vi "OE2012&OE2022_Configure Auxout.vi"(7 "OE2012&OE2022_\nConfigure Auxout":T1={"Offset(%)"=0.0, "Expand"=1, "Source"=3, "Aux Output"=1, "Sensitivity "=24, "DC Voltage"=0.0} {"DC Voltage" min=-100.0 max=100.0 format="%#.2g"; "Sensitivity" items=["1 nV/fA", "2 nV/fA", "5 nV/fA", "10 nV/fA", "20 nV/fA", "50 nV/fA", "100 nV/fA", "200 nV/fA", "500 nV/fA", "1 uV/pA", "2 uV/pA", "5 uV/pA", "10 uV/pA", "20 uV/pA", "50 uV/pA", "100 uV/pA", "200 uV/pA", "500 uV/pA", "1 mV/nA", "2 mV/nA", "5 mV/nA", "10 mV/nA", "20 mV/nA", "50 mV/nA", "100 mV/nA", "200 mV/nA", "500 mV/nA", "1 V/uA", "2 V/uA", "5 V/uA"]; "Aux Output" items=["AUX1"=1, "AUX2"=2, "AUX3"=3, "AUX4"=4]; "Source" items=["DC OUT", "X-Demod1", "Y-Demod1", "R-Demod1", "Theta-Demod1", "X-Demod2", "Y-Demod2", "R-Demod2", "Theta-Demod2", "X-Demod3", "Y-Demod3", "R-Demod3", "Theta-Demod3", "X-Demod4", "Y-Demod4", "R-Demod4", "Theta-Demod4", "X-Demod5", "Y-Demod5", "R-Demod5", "Theta-Demod5", "X-Demod6", "Y-Demod6", "R-Demod6", "Theta-Demod6", "X-Demod7", "Y-Demod7", "R-Demod7", "Theta-Demod7", "X-Demod8", "Y-Demod8", "R-Demod8", "Theta-Demod8", "AUXIN1", "AUXIN2", "AUXIN3", "AUXIN4"]; "Expand" min=1 max=256; "Offset(%)" min=-100.0 max=100.0 format="%#.2g"}, 8 "Error in (no error)":errorcluster caption="error out（no error）", 9 "Remote Mode":u16(ring) items=["USB", "RS232", "GPIB", "Ethernet"], 11 "VISA resource name":refnum<visa-resource-name>) -> (0 "Error out":errorcluster caption="error out", 1 "Output String":string, 3 "VISA resource  out":refnum<visa-resource-name>)   [LabVIEW 2011]
panel:
  out "Connection ID out":refnum<k5>
  in  "Connection ID in":refnum<k5>
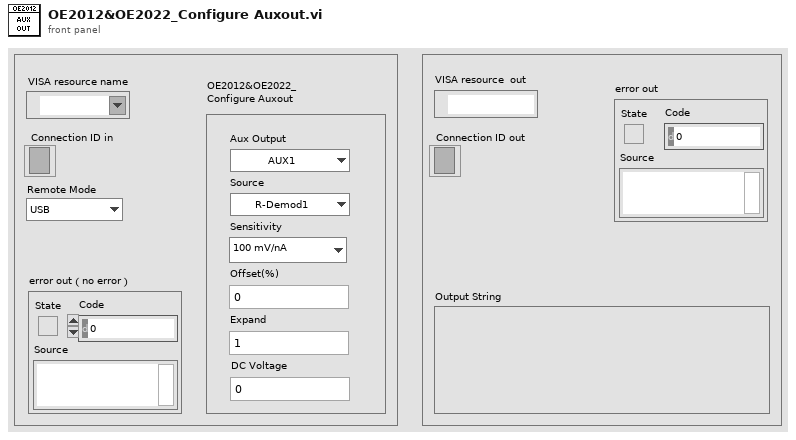
[diagram p1: front panel]
types:
  T1 = cluster{"Offset(%)":dbl, "Expand":i16, "Source":u16, "Aux Output":u16, "Sensitivity ":u16, "DC Voltage":dbl}
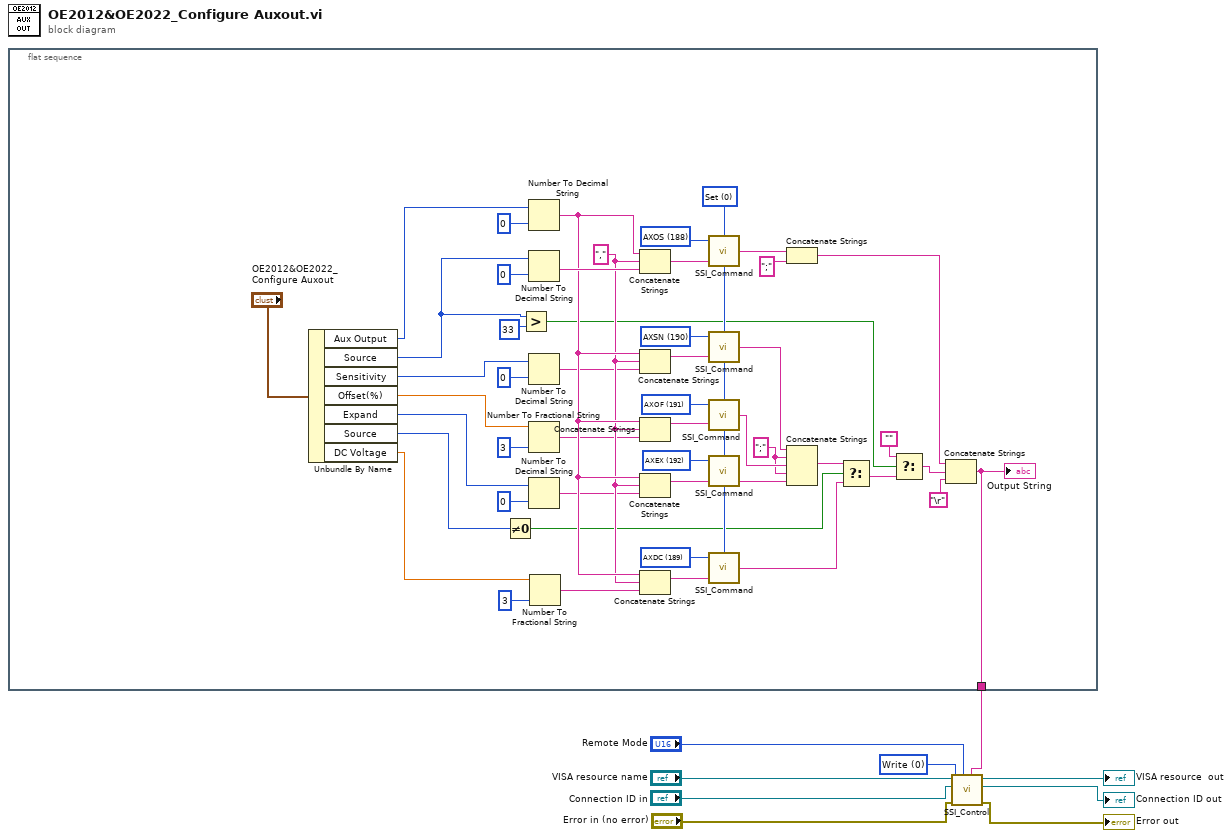
[diagram p0: block diagram]
diagram:
  w8 = u16 0 items=["Write", "Read"] ("Control")
  n1 = flat-sequence {
    tunnel: [w22] -> w1
    frame #0 {
      w10 = u16 189 items=["ISRC", "IGND", "ICPL", "ILIN", "PHAS", "FMOD", "RSLP", "FREQ", "SWPT", "SLLM", "SULM", "SSLL", "SSLG", "STLM", "SWRM", "IRNG", "SENS", "RMOD", "OFLT", "OFSL", "SYNC", "DMOD", "HARM", "DARB", "SWVT", "SLVL", "SVLL", "SVUL", "SVSL", "SVSG", "SVTM", "SVRM", "RALL", "SNAP", "OUTP", "OAUX", "COUT", "CAUX", "COFP", "CEXP", "FPOP", "OEXP", "*IDN", "*RST", "OVLD", "INOV", "GNOV", "*PLL", "SSET", "RSET", "AGAN", "APHS", "ARSV", "ASCL", "EQCD", "EQCS", "SPED", "SRAT", "SLEN", "SSLE", "STRG", "SPRM", "STRD", "PAUS", "REST", "SPTS", "TRCA", "TEMP", "RSTU", "INHZ", "DEQU", "SADD", "ARNG", "CSPE", "ISRCD", "IGNDD", "ICPLD", "ILIND", "PHASD", "FMODD", "RSLPD", "FREQD", "SWPTD", "SLLMD", "SULMD", "SSLLD", "SSLGD", "STLMD", "SWRMD", "SENSD", "RMODD", "OFLTD", "OFSLD", "SYNCD", "HARMD", "EQCDD", "EQCSD", "SNAPD", "OUTPD", "SWVTD", "SLVLD", "SVLLD", "SVULD", "SVSLD", "SVSGD", "SVTMD", "SVRMD", "SVDCD", "ARSVD", "AGAND", "APHSD", "ASCLD", "FPOPD", "CAUXD", "OEXPD", "SPEDD", "SRATD", "SLEND", "SSLED", "STRGD", "SPRMD", "STRDD", "PAUSD", "RESTD", "SPTSD", "TRCAD", "*IDND", "*RSTD", "INOVD", "GNOVD", "*PLLD", "SSETD", "RSETD", "RALLD", "NIPA", "NSMA", "NGWA", "NMAC", "NMOD", "TRIG", "TRCB", "INHZD", "ISAMD", "IRAGD", "RRAGD", "SOFFD", "DMODD", "COUTD", "COFPD", "CEXPD", "ARNGD", "OAUXD", "TRIM", "SUITD", "SNHZD", "AOFSD", "RSRC", "FEXT", "FINT", "DSRC", "DARF", "DEAF", "DREF", "SSRC", "STTL", "SIGO", "SLVL", "SOFF", "SPHS", "TPHS", "SMOD", "MARF", "AMSR", "AMDP", "FMSR", "FMDV", "PMSR", "PMDV", "CHDC", "AUXV", "AFLT", "AOFP", "DSELD", "FEMSD", "SLVTD", "SLVBD", "DMFR", "FCMB", "AXOS", "AXDC", "AXSN", "AXOF", "AXEX"] ("Command Type")
      w11 = u16 192 items=["ISRC", "IGND", "ICPL", "ILIN", "PHAS", "FMOD", "RSLP", "FREQ", "SWPT", "SLLM", "SULM", "SSLL", "SSLG", "STLM", "SWRM", "IRNG", "SENS", "RMOD", "OFLT", "OFSL", "SYNC", "DMOD", "HARM", "DARB", "SWVT", "SLVL", "SVLL", "SVUL", "SVSL", "SVSG", "SVTM", "SVRM", "RALL", "SNAP", "OUTP", "OAUX", "COUT", "CAUX", "COFP", "CEXP", "FPOP", "OEXP", "*IDN", "*RST", "OVLD", "INOV", "GNOV", "*PLL", "SSET", "RSET", "AGAN", "APHS", "ARSV", "ASCL", "EQCD", "EQCS", "SPED", "SRAT", "SLEN", "SSLE", "STRG", "SPRM", "STRD", "PAUS", "REST", "SPTS", "TRCA", "TEMP", "RSTU", "INHZ", "DEQU", "SADD", "ARNG", "CSPE", "ISRCD", "IGNDD", "ICPLD", "ILIND", "PHASD", "FMODD", "RSLPD", "FREQD", "SWPTD", "SLLMD", "SULMD", "SSLLD", "SSLGD", "STLMD", "SWRMD", "SENSD", "RMODD", "OFLTD", "OFSLD", "SYNCD", "HARMD", "EQCDD", "EQCSD", "SNAPD", "OUTPD", "SWVTD", "SLVLD", "SVLLD", "SVULD", "SVSLD", "SVSGD", "SVTMD", "SVRMD", "SVDCD", "ARSVD", "AGAND", "APHSD", "ASCLD", "FPOPD", "CAUXD", "OEXPD", "SPEDD", "SRATD", "SLEND", "SSLED", "STRGD", "SPRMD", "STRDD", "PAUSD", "RESTD", "SPTSD", "TRCAD", "*IDND", "*RSTD", "INOVD", "GNOVD", "*PLLD", "SSETD", "RSETD", "RALLD", "NIPA", "NSMA", "NGWA", "NMAC", "NMOD", "TRIG", "TRCB", "INHZD", "ISAMD", "IRAGD", "RRAGD", "SOFFD", "DMODD", "COUTD", "COFPD", "CEXPD", "ARNGD", "OAUXD", "TRIM", "SUITD", "SNHZD", "AOFSD", "RSRC", "FEXT", "FINT", "DSRC", "DARF", "DEAF", "DREF", "SSRC", "STTL", "SIGO", "SLVL", "SOFF", "SPHS", "TPHS", "SMOD", "MARF", "AMSR", "AMDP", "FMSR", "FMDV", "PMSR", "PMDV", "CHDC", "AUXV", "AFLT", "AOFP", "DSELD", "FEMSD", "SLVTD", "SLVBD", "DMFR", "FCMB", "AXOS", "AXDC", "AXSN", "AXOF", "AXEX"] ("Command Type")
      w12 = u16 191 items=["ISRC", "IGND", "ICPL", "ILIN", "PHAS", "FMOD", "RSLP", "FREQ", "SWPT", "SLLM", "SULM", "SSLL", "SSLG", "STLM", "SWRM", "IRNG", "SENS", "RMOD", "OFLT", "OFSL", "SYNC", "DMOD", "HARM", "DARB", "SWVT", "SLVL", "SVLL", "SVUL", "SVSL", "SVSG", "SVTM", "SVRM", "RALL", "SNAP", "OUTP", "OAUX", "COUT", "CAUX", "COFP", "CEXP", "FPOP", "OEXP", "*IDN", "*RST", "OVLD", "INOV", "GNOV", "*PLL", "SSET", "RSET", "AGAN", "APHS", "ARSV", "ASCL", "EQCD", "EQCS", "SPED", "SRAT", "SLEN", "SSLE", "STRG", "SPRM", "STRD", "PAUS", "REST", "SPTS", "TRCA", "TEMP", "RSTU", "INHZ", "DEQU", "SADD", "ARNG", "CSPE", "ISRCD", "IGNDD", "ICPLD", "ILIND", "PHASD", "FMODD", "RSLPD", "FREQD", "SWPTD", "SLLMD", "SULMD", "SSLLD", "SSLGD", "STLMD", "SWRMD", "SENSD", "RMODD", "OFLTD", "OFSLD", "SYNCD", "HARMD", "EQCDD", "EQCSD", "SNAPD", "OUTPD", "SWVTD", "SLVLD", "SVLLD", "SVULD", "SVSLD", "SVSGD", "SVTMD", "SVRMD", "SVDCD", "ARSVD", "AGAND", "APHSD", "ASCLD", "FPOPD", "CAUXD", "OEXPD", "SPEDD", "SRATD", "SLEND", "SSLED", "STRGD", "SPRMD", "STRDD", "PAUSD", "RESTD", "SPTSD", "TRCAD", "*IDND", "*RSTD", "INOVD", "GNOVD", "*PLLD", "SSETD", "RSETD", "RALLD", "NIPA", "NSMA", "NGWA", "NMAC", "NMOD", "TRIG", "TRCB", "INHZD", "ISAMD", "IRAGD", "RRAGD", "SOFFD", "DMODD", "COUTD", "COFPD", "CEXPD", "ARNGD", "OAUXD", "TRIM", "SUITD", "SNHZD", "AOFSD", "RSRC", "FEXT", "FINT", "DSRC", "DARF", "DEAF", "DREF", "SSRC", "STTL", "SIGO", "SLVL", "SOFF", "SPHS", "TPHS", "SMOD", "MARF", "AMSR", "AMDP", "FMSR", "FMDV", "PMSR", "PMDV", "CHDC", "AUXV", "AFLT", "AOFP", "DSELD", "FEMSD", "SLVTD", "SLVBD", "DMFR", "FCMB", "AXOS", "AXDC", "AXSN", "AXOF", "AXEX"] ("Command Type")
      w13 = u16 190 items=["ISRC", "IGND", "ICPL", "ILIN", "PHAS", "FMOD", "RSLP", "FREQ", "SWPT", "SLLM", "SULM", "SSLL", "SSLG", "STLM", "SWRM", "IRNG", "SENS", "RMOD", "OFLT", "OFSL", "SYNC", "DMOD", "HARM", "DARB", "SWVT", "SLVL", "SVLL", "SVUL", "SVSL", "SVSG", "SVTM", "SVRM", "RALL", "SNAP", "OUTP", "OAUX", "COUT", "CAUX", "COFP", "CEXP", "FPOP", "OEXP", "*IDN", "*RST", "OVLD", "INOV", "GNOV", "*PLL", "SSET", "RSET", "AGAN", "APHS", "ARSV", "ASCL", "EQCD", "EQCS", "SPED", "SRAT", "SLEN", "SSLE", "STRG", "SPRM", "STRD", "PAUS", "REST", "SPTS", "TRCA", "TEMP", "RSTU", "INHZ", "DEQU", "SADD", "ARNG", "CSPE", "ISRCD", "IGNDD", "ICPLD", "ILIND", "PHASD", "FMODD", "RSLPD", "FREQD", "SWPTD", "SLLMD", "SULMD", "SSLLD", "SSLGD", "STLMD", "SWRMD", "SENSD", "RMODD", "OFLTD", "OFSLD", "SYNCD", "HARMD", "EQCDD", "EQCSD", "SNAPD", "OUTPD", "SWVTD", "SLVLD", "SVLLD", "SVULD", "SVSLD", "SVSGD", "SVTMD", "SVRMD", "SVDCD", "ARSVD", "AGAND", "APHSD", "ASCLD", "FPOPD", "CAUXD", "OEXPD", "SPEDD", "SRATD", "SLEND", "SSLED", "STRGD", "SPRMD", "STRDD", "PAUSD", "RESTD", "SPTSD", "TRCAD", "*IDND", "*RSTD", "INOVD", "GNOVD", "*PLLD", "SSETD", "RSETD", "RALLD", "NIPA", "NSMA", "NGWA", "NMAC", "NMOD", "TRIG", "TRCB", "INHZD", "ISAMD", "IRAGD", "RRAGD", "SOFFD", "DMODD", "COUTD", "COFPD", "CEXPD", "ARNGD", "OAUXD", "TRIM", "SUITD", "SNHZD", "AOFSD", "RSRC", "FEXT", "FINT", "DSRC", "DARF", "DEAF", "DREF", "SSRC", "STTL", "SIGO", "SLVL", "SOFF", "SPHS", "TPHS", "SMOD", "MARF", "AMSR", "AMDP", "FMSR", "FMDV", "PMSR", "PMDV", "CHDC", "AUXV", "AFLT", "AOFP", "DSELD", "FEMSD", "SLVTD", "SLVBD", "DMFR", "FCMB", "AXOS", "AXDC", "AXSN", "AXOF", "AXEX"] ("Command Type")
      w14 = u16 188 items=["ISRC", "IGND", "ICPL", "ILIN", "PHAS", "FMOD", "RSLP", "FREQ", "SWPT", "SLLM", "SULM", "SSLL", "SSLG", "STLM", "SWRM", "IRNG", "SENS", "RMOD", "OFLT", "OFSL", "SYNC", "DMOD", "HARM", "DARB", "SWVT", "SLVL", "SVLL", "SVUL", "SVSL", "SVSG", "SVTM", "SVRM", "RALL", "SNAP", "OUTP", "OAUX", "COUT", "CAUX", "COFP", "CEXP", "FPOP", "OEXP", "*IDN", "*RST", "OVLD", "INOV", "GNOV", "*PLL", "SSET", "RSET", "AGAN", "APHS", "ARSV", "ASCL", "EQCD", "EQCS", "SPED", "SRAT", "SLEN", "SSLE", "STRG", "SPRM", "STRD", "PAUS", "REST", "SPTS", "TRCA", "TEMP", "RSTU", "INHZ", "DEQU", "SADD", "ARNG", "CSPE", "ISRCD", "IGNDD", "ICPLD", "ILIND", "PHASD", "FMODD", "RSLPD", "FREQD", "SWPTD", "SLLMD", "SULMD", "SSLLD", "SSLGD", "STLMD", "SWRMD", "SENSD", "RMODD", "OFLTD", "OFSLD", "SYNCD", "HARMD", "EQCDD", "EQCSD", "SNAPD", "OUTPD", "SWVTD", "SLVLD", "SVLLD", "SVULD", "SVSLD", "SVSGD", "SVTMD", "SVRMD", "SVDCD", "ARSVD", "AGAND", "APHSD", "ASCLD", "FPOPD", "CAUXD", "OEXPD", "SPEDD", "SRATD", "SLEND", "SSLED", "STRGD", "SPRMD", "STRDD", "PAUSD", "RESTD", "SPTSD", "TRCAD", "*IDND", "*RSTD", "INOVD", "GNOVD", "*PLLD", "SSETD", "RSETD", "RALLD", "NIPA", "NSMA", "NGWA", "NMAC", "NMOD", "TRIG", "TRCB", "INHZD", "ISAMD", "IRAGD", "RRAGD", "SOFFD", "DMODD", "COUTD", "COFPD", "CEXPD", "ARNGD", "OAUXD", "TRIM", "SUITD", "SNHZD", "AOFSD", "RSRC", "FEXT", "FINT", "DSRC", "DARF", "DEAF", "DREF", "SSRC", "STTL", "SIGO", "SLVL", "SOFF", "SPHS", "TPHS", "SMOD", "MARF", "AMSR", "AMDP", "FMSR", "FMDV", "PMSR", "PMDV", "CHDC", "AUXV", "AFLT", "AOFP", "DSELD", "FEMSD", "SLVTD", "SLVBD", "DMFR", "FCMB", "AXOS", "AXDC", "AXSN", "AXOF", "AXEX"] ("Command Type")
      w29 = ";" ("替换字符串(\"\")")
      w46 = "," ("字符串")
      w51 = u16 0 items=["Set", "Query"] ("Opera")
      n2 = Unbundle By Name("OE2012&OE2022_\nConfigure Auxout") -> ("Aux Output"=w21:u16, "Source"=w19:u16, "Sensitivity"=w20:u16, "Offset(%)"=w18:dbl, "Expand"=w17:i16, "Source"=w16:u16, "DC Voltage"=w15:dbl)
      n3 = Not Equal To 0?(x=w16) -> (x != 0?=w32:bool)
      n4 = Greater?(x=w19, y=u16 33) -> (0:w25:bool)
      n5 = Number To Decimal String(number=w21, width (-)=i16 0 ("精度(6)")) -> (decimal integer string=w47:string)
      n6 = Number To Decimal String(number=w19, width (-)=i16 0 ("精度(6)")) -> (decimal integer string=w54:string)
      n7 = Number To Decimal String(number=w20, width (-)=i16 0 ("精度(6)")) -> (decimal integer string=w33:string)
      n8 = Number To Fractional String(number=w18, precision (6)=i16 3 ("精度(6)")) -> (F-format string=w38:string)  [unwired: 2 in]
      n9 = Number To Decimal String(number=w17, width (-)=i16 0 ("精度(6)")) -> (decimal integer string=w37:string)
      n10 = Number To Fractional String(number=w15, precision (6)=i16 3 ("精度(6)")) -> (F-format string=w34:string)  [unwired: 2 in]
      n11 = Concatenate Strings(w47, w46, w54) -> (w53:string)
      n12 = Concatenate Strings(w47, w46, w33) -> (w41:string)
      n13 = Concatenate Strings(w47, w46, w38) -> (w40:string)
      n14 = Concatenate Strings(w47, w46, w37) -> (w39:string)
      n15 = Concatenate Strings(w47, w46, w34) -> (w35:string)
      n16 = call "SSI_Command.vi"("Opera"=w51, "Paramter"=w53, "Command Type"=w14) -> ("Output string"=w55:string)  [unwired: 1 in]
      n17 = call "SSI_Command.vi"("Opera"=w51, "Paramter"=w41, "Command Type"=w13) -> ("Output string"=w31:string)  [unwired: 1 in]
      n18 = call "SSI_Command.vi"("Opera"=w51, "Paramter"=w40, "Command Type"=w12) -> ("Output string"=w30:string)  [unwired: 1 in]
      n19 = call "SSI_Command.vi"("Opera"=w51, "Paramter"=w39, "Command Type"=w11) -> ("Output string"=w43:string)  [unwired: 1 in]
      n20 = call "SSI_Command.vi"("Opera"=w51, "Paramter"=w35, "Command Type"=w10) -> ("Output string"=w27:string)  [unwired: 1 in]
      n21 = Concatenate Strings(w55, ";" ("替换字符串(\"\")")) -> (w50:string)
      n22 = Concatenate Strings(w31, w29, w30, w29, w43) -> (w28:string)
      n23 = Select(t=w28, s=w32, f=w27) -> (s? t:f=w26:string)
      n24 = Select(t="", s=w25, f=w26) -> (s? t:f=w23:string)
      n25 = Concatenate Strings(w50, w23, "\r") -> (w22:string)
      "Output String" <- w22
    }
  }
  n26 = call "SSI_Control.vi"("Write Buffer"=w1, "Remote Mode"="Remote Mode", "Error in (no error)"="Error in (no error)", "Control"=w8, "Connection ID in"="Connection ID in", "VISA resource name"="VISA resource name") -> ("Error out"=→"Error out":errorcluster, "Connection ID out"=→"Connection ID out":refnum<k5>, "VISA resource  out"=→"VISA resource  out":refnum<visa-resource-name>)  [unwired: 2 in, 1 out]
